vi "DigitalRead_MultiTask.vi"(2 "error in":errorcluster, 3 "mutiTask":refnum<k21>) -> (0 "error out":errorcluster, 1 "read":bool[](array[boolean]))   [LabVIEW 2015]
uses:
  <vilib>/DAQmx/read.llb/DAQmx Read (Digital 1D Bool NChan 1Samp 1Line).vi
  <vilib>/DAQmx/miscellaneous.llb/DAQmx Fill In Error Info.vi
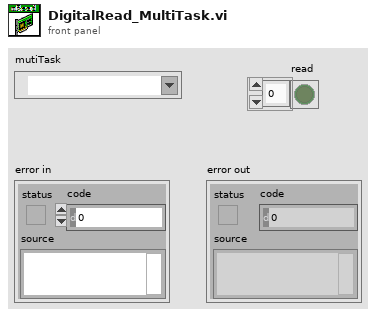
[diagram p1: front panel]
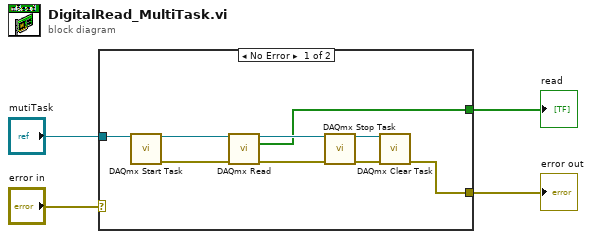
[diagram p0: block diagram]
diagram:
  n1 = case shown="No Error" "error in" {
    selector: "error in" -> [_ w14]
    tunnel: "mutiTask" -> [w7 _]
    tunnel: [w6 w14] -> w2
    tunnel: [w5 _] -> w1
    frame No Error {
      n2 = call <vilib>:"DAQmx Start Task.vi"("task/channels in"=w7) -> ("task out"=w13:refnum<k21>, "error out"=w12:errorcluster)  [unwired: 13 in]
      n3 = call-poly <vilib>:"DAQmx Read.vi"("task/channels in"=w13, "error in"=w12) -> ("task out"=w11:refnum<k21>, "data"=w5:bool[], "error out"=w10:errorcluster)  [unwired: 11 in]
      n4 = call <vilib>:"DAQmx Stop Task.vi"("task/channels in"=w11, "error in"=w10) -> ("task out"=w8:refnum<k21>, "error out"=w9:errorcluster)  [unwired: 12 in]
      n5 = call <vilib>:"DAQmx Clear Task.vi"("task in"=w8, "error in"=w9) -> ("error out"=w6:errorcluster)  [unwired: 13 in]
    }
    frame Error {
    }
  }
  "error out" <- w2
  "read" <- w1
